vi "Move rel mMc Edited.vi"(5 "Controller #":string, 6 "rev dir?":bool, 7 "Port In":T1, 8 "error in (no error)":errorcluster, 11 "pos incr":dbl) -> (0 "error out":errorcluster, 3 "Port Out":T1)   [LabVIEW 2021]
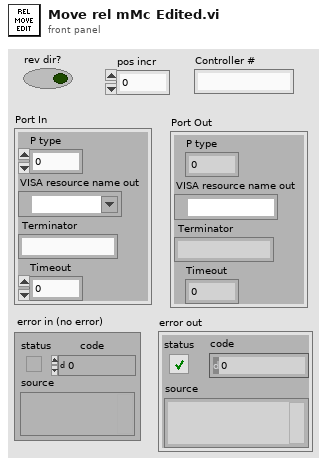
[diagram p1: front panel]
types:
  T1 = cluster{"P type":u16, "VISA resource name out":refnum<visa-resource-name>, " Terminator":string, "Timeout":i32}
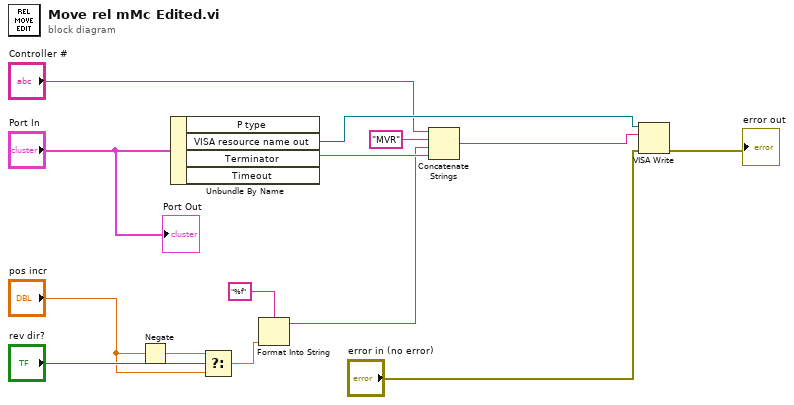
[diagram p0: block diagram]
diagram:
  n1 = Negate(x="pos incr") -> (-x=w3:dbl)
  n2 = Unbundle By Name("Port In") -> ("VISA resource name out"=w12:refnum<visa-resource-name>, "Terminator"=w9:string)  [unwired: 2 out]
  n3 = Select(t=w3, s="rev dir?", f="pos incr") -> (s? t:f=w2:dbl)
  n4 = Format Into String(format string="%f", w2) -> (resulting string=w8:string)  [unwired: 2 in, 1 out]
  n5 = Concatenate Strings("Controller #", "MVR" ("string"), w8, w9) -> (w1:string)
  n6 = VISA Write(VISA resource name=w12, write buffer=w1, error in (no error)="error in (no error)") -> (error out=→"error out":errorcluster)  [unwired: 2 out]
  "Port Out" <- "Port In"
